vi "run.vi"(8 "error in (no error)":errorcluster, 11 "M1M3SAL in":refnum<class "M1M3SAL.lvclass">) -> (0 "error out":errorcluster, 3 "M1M3SAL out":refnum<class "M1M3SAL.lvclass">)   [LabVIEW 2016, in "M1M3SupportCommunicator.lvlib" / "M1M3SAL.lvclass"]
uses:
  M1M3SAL.lvclass
  M1M3SAL.lvclass/M1M3SAL.ctl
  UserEvents/UserEvents.lvclass/UserEvents.ctl
  DataTypes/Topics/EventSummaryState.ctl
  DataTypes/Topics/Parts/Timestamp.ctl
  DataTypes/Topics/Parts/SummaryStates.ctl
  DataTypes/Topics/Parts/CommandId.ctl
  DataTypes/Topics/CommandStart.ctl
  Commands/StartCommand/StartCommand.lvclass
  D:/Code/ts_M1M3Support/Commands/Command/Command.lvclass
  DataTypes/General/ProcessCommandEvent.ctl
  Commands/Command/Command.lvclass
  Commands/StartCommand/StartCommand.lvclass/StartCommand.ctl
  DataTypes/Topics/CommandEnable.ctl
  Commands/EnableCommand/EnableCommand.lvclass
  Commands/EnableCommand/EnableCommand.lvclass/EnableCommand.ctl
  DataTypes/Topics/CommandDisable.ctl
  Commands/DisableCommand/DisableCommand.lvclass
  Commands/DisableCommand/DisableCommand.lvclass/DisableCommand.ctl
  DataTypes/Topics/CommandStandby.ctl
  Commands/StandbyCommand/StandbyCommand.lvclass
  Commands/StandbyCommand/StandbyCommand.lvclass/StandbyCommand.ctl
  DataTypes/Topics/CommandExit.ctl
  Commands/ExitCommand/ExitCommand.lvclass
  Commands/ExitCommand/ExitCommand.lvclass/ExitCommand.ctl
  DataTypes/Topics/M1M3SupportTopics.lvlib
  DataTypes/General/M1M3SupportGeneral.lvlib
  UserEvents/UserEvents.lvclass
panel:
  out "Shutdown":bool
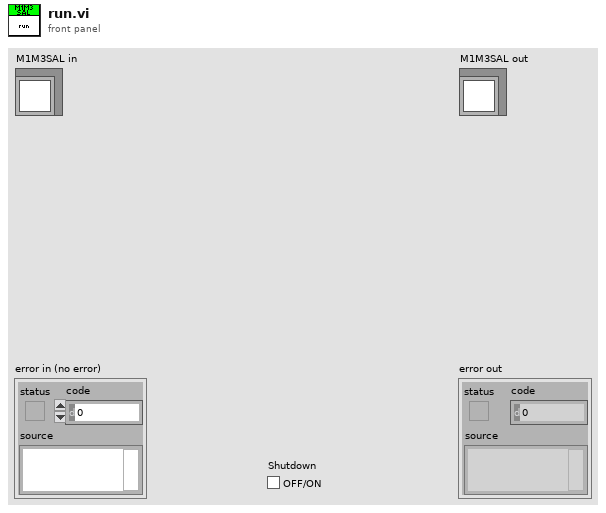
[diagram p1: front panel]
types:
  T1 = typedef "M1M3SupportTopics.lvlib/EventSummaryState.ctl" = cluster{"Timestamp":T2, "SummaryStates":T3}
  T2 = typedef "M1M3SupportTopics.lvlib/Timestamp.ctl" = dbl
  T3 = typedef "M1M3SupportTopics.lvlib/SummaryStates.ctl" = enum16{"OfflineState", "StandbyState", "DisabledState", "EnabledState", "FaultState"}
  T4 = typedef "M1M3SupportTopics.lvlib/CommandId.ctl" = i32
  T5 = typedef "M1M3SupportGeneral.lvlib/ProcessCommandEvent.ctl" = cluster{"Command":refnum<class "Command.lvclass">}
  T6 = typedef "M1M3SupportTopics.lvlib/CommandStart.ctl" = cluster{"CommandId":T4, "Start":bool, "SettingToApply":string}
  T7 = typedef "M1M3SupportTopics.lvlib/CommandEnable.ctl" = cluster{"CommandId":T4, "Enable":bool}
  T8 = typedef "M1M3SupportTopics.lvlib/CommandDisable.ctl" = cluster{"CommandId":T4, "Disable":bool}
  T9 = typedef "M1M3SupportTopics.lvlib/CommandStandby.ctl" = cluster{"CommandId":T4, "Standby":bool}
  T10 = typedef "M1M3SupportTopics.lvlib/CommandExit.ctl" = cluster{"CommandId":T4, "Exit":bool}
  T11 = typedef "M1M3SupportCommunicator.lvlib/Message.ctl" = cluster{"Header":T12, "Data":variant}
  T12 = typedef "M1M3SupportCommunicator.lvlib/MessageHeader.ctl" = cluster{"Type":T13, "Topic":T14, "Size":i32}
  T13 = typedef "M1M3SupportCommunicator.lvlib/MessageTypes.ctl" = enum8{"None", "PutSample", "GetNextSample", "LogEvent", "GetEvent", "IssueCommand", "CommandId", "WaitForCompletion", "AcceptCommand", "AckCommand"}
  T14 = typedef "M1M3SupportCommunicator.lvlib/MessageTopics.ctl" = enum8{"None", "ForceActuatorData", "MirrorForceData", "HardpointData", "AirData", "DynamicData", "FPGAData", "IMSData", "ForceActuatorStatus", "ElevationData", "HardpointStatus", "HardpointActuatorChase", "AirStatus", "ForceActuatorSafetyChecks", "ForceActuatorTest", "ActuatorBroadcastCounter", "StatusChecks", "CellChecks", "HardpointActuatorBreakaway", "RaiseMirrorComplete", "ILCCommunication", "ElevationAngleChecks", "DetailedState", "ServoLoops", "ForceActuatorInfo", "LowerMirrorComplete", "HardpointActuatorInfo", "SettingsApplied", "ErrorCode", "StartupChecks", "SummaryState", "SettingVersions", "ActuatorTestStatus", "AppliedSettingsMatchStart", "Enable", "EnterMaintenance", "Standby", "AbortLowerM1M3", "ApplyAberrationByForces", "ApplyAOSCorrectionByBendingModes", "ClearAOSCorrection", "Start", "RaiseM1M3", "TestForceActuator", "LowerM1M3", "ApplyAOSCorrectionByForces", "Disable", "ApplyAberationByBendingMode", "TestHardpoint", "ManipulateM1M3", "ClearAberration", "Exit", "TestAir", "AbortRaiseM1M3", "MoveHardpointActuators", "ExitMaintenance", "Shutdown"}
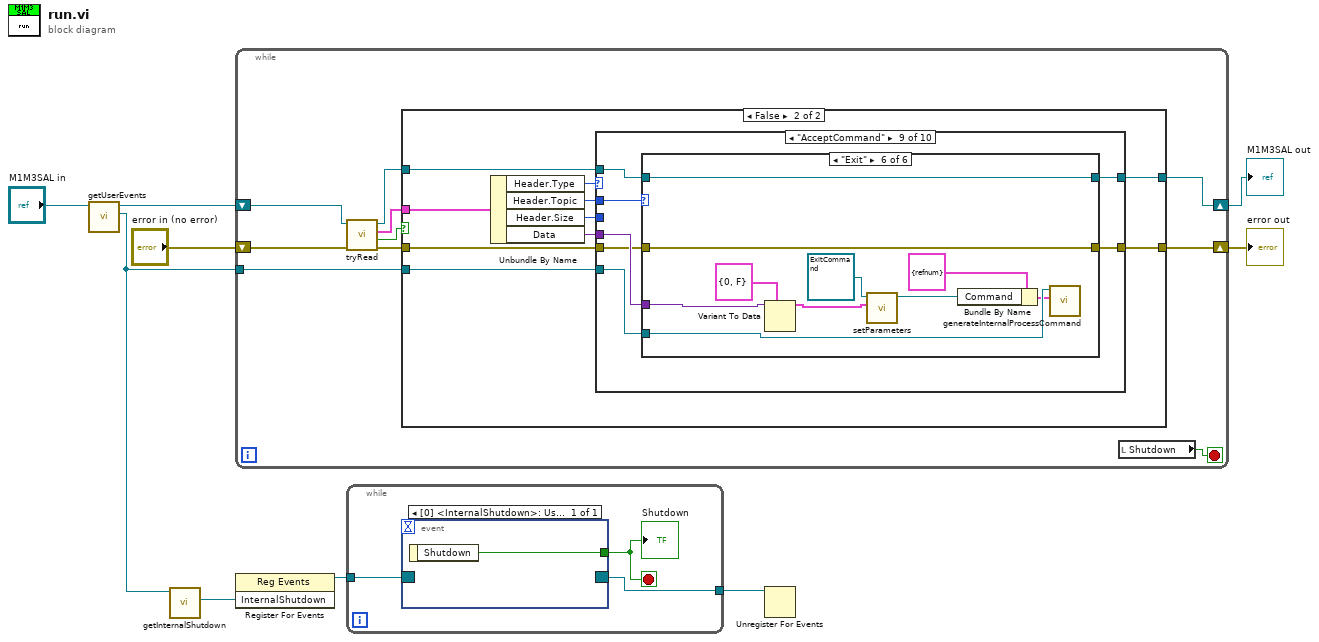
[diagram p0: block diagram]
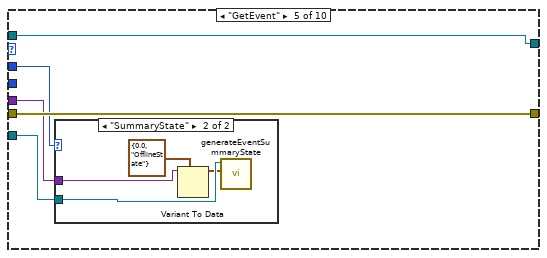
[diagram p7: hidden frame]
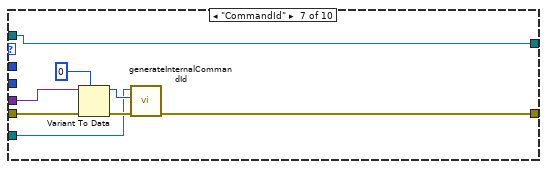
[diagram p10: hidden frame]
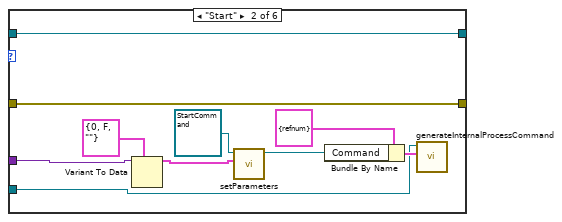
[diagram p13: hidden frame]
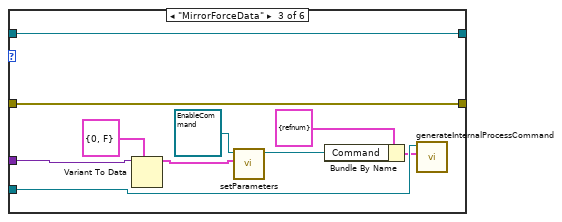
[diagram p14: hidden frame]
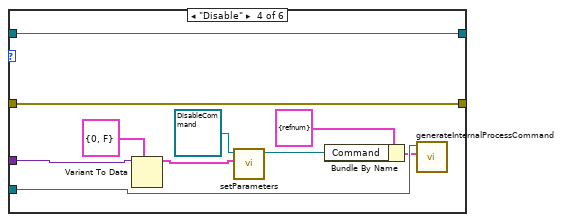
[diagram p15: hidden frame]
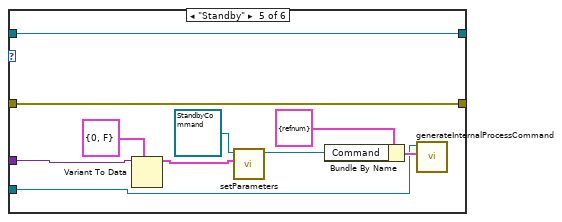
[diagram p16: hidden frame]
diagram:
  n1 = call "getUserEvents.vi"("M1M3SAL in"="M1M3SAL in") -> ("UserEvents"=w4:refnum<class "UserEvents.lvclass">, "M1M3SAL out"=w8:refnum<class "M1M3SAL.lvclass">)  [unwired: 9 in]
  n2 = call "getInternalShutdown.vi"("UserEvents in"=w4) -> ("InternalShutdown"=w3:refnum<user-event>)  [unwired: 9 in, 1 out]
  n3 = while {
    tunnel: w4 -> [w18]
    shift-right: [w15] -> w6
    shift-left: w8 -> [w17]
    shift-right: [w14] -> w5
    shift-left: "error in (no error)" -> [w13]
    stop <- w11 stop-if-true
    n4 = call "tryRead.vi"("error in (no error)"=w13, "M1M3SAL in"=w17) -> ("error out"=w12:errorcluster, "Timeout"=w10:bool, "Message"=w19:T11, "M1M3SAL out"=w16:refnum<class "M1M3SAL.lvclass">)  [unwired: 6 in]
    n5 = case shown="False" w10 {
      tunnel: w19 -> [_ w31]
      tunnel: w18 -> [_ w26]
      tunnel: w16 -> [w21 w25]
      tunnel: [w21 w24] -> w15
      tunnel: [w20 w23] -> w14
      tunnel: w12 -> [w20 w22]
      frame True {
      }
      frame False {
        n6 = Unbundle By Name(w31) -> ("Header.Type"=w30:T13, "Header.Topic"=w27:T14, "Header.Size"=w28:i32, "Data"=w29:variant)
        n7 = case shown="\"AcceptCommand\"" w30 {
          tunnel: w29 -> [_ _ _ _ w40 _ w57 _ w66 _]
          tunnel: w28 -> [_ _ _ _ _ _ _ _ _ _]
          tunnel: w27 -> [_ _ _ _ w41 _ _ _ w67 _]
          tunnel: w26 -> [_ _ _ _ w42 _ w51 _ w65 _]
          tunnel: w25 -> [w33 w35 w37 w39 w44 w50 w56 w60 w61 w121]
          tunnel: [w33 w35 w37 w39 w44 w50 w56 w60 w62 w121] -> w24
          tunnel: w22 -> [w32 w34 w36 w38 w43 w49 w55 w59 w64 w120]
          tunnel: [w32 w34 w36 w38 w43 w49 w52 w59 w63 w120] -> w23
          frame "None", Default {
          }
          frame "PutSample" {
          }
          frame "GetNextSample" {
          }
          frame "LogEvent" {
          }
          frame "GetEvent" {
            n8 = case shown="\"SummaryState\"" w41 {
              tunnel: w42 -> [_ w46]
              tunnel: w40 -> [_ w48]
              frame "None", Default {
              }
              frame "SummaryState" {
                n9 = Variant To Data(type=T1 {"Timestamp"=0.0, "SummaryStates"=enum."OfflineState"} ("EventSummaryState"), Variant=w48) -> (data=w45:T1)  [unwired: 1 in, 1 out]
                n10 = call "generateEventSummaryState.vi"("EventSummaryState"=w45, "UserEvents in"=w46) -> ()  [unwired: 8 in, 2 out]
              }
            }
          }
          frame "IssueCommand" {
          }
          frame "CommandId" {
            n11 = Variant To Data(error in=w55, type=T4 0 ("CommandId"), Variant=w57) -> (data=w54:T4, error out=w53:errorcluster)
            n12 = call "generateInternalCommandId.vi"("error in (no error)"=w53, "CommandId"=w54, "UserEvents in"=w51) -> ("error out"=w52:errorcluster)  [unwired: 7 in, 1 out]
          }
          frame "WaitForCompletion" {
          }
          frame "AcceptCommand" {
            n13 = case shown="\"Exit\"" w67 {
              tunnel: w66 -> [_ w79 w89 w99 w109 w119]
              tunnel: w65 -> [_ w70 w81 w91 w100 w111]
              tunnel: w64 -> [w69 w76 w86 w96 w106 w116]
              tunnel: [w69 w76 w86 w96 w106 w116] -> w63
              tunnel: [w68 w75 w85 w95 w105 w115] -> w62
              tunnel: w61 -> [w68 w75 w85 w95 w105 w115]
              frame "None", Default {
              }
              frame "Start" {
                n14 = Variant To Data(type=T6 {"CommandId"=0, "Start"=FALSE, "SettingToApply"=""} ("CommandStart"), Variant=w79) -> (data=w73:T6)  [unwired: 1 in, 1 out]
                n15 = call "setParameters.vi"("Parameters"=w73, "StartCommand in"=refnum<class "StartCommand.lvclass"> refnum ("StartCommand.lvclass")) -> ("StartCommand out"=w72:refnum<class "StartCommand.lvclass">)  [unwired: 9 in]
                n16 = Bundle By Name(cluster=T5 {"Command"=refnum} ("ProcessCommandEvent"), "Command"=w72) -> (w71:T5)
                n17 = call "generateInternalProcessCommand.vi"("ProcessCommandEvent"=w71, "UserEvents in"=w70) -> ()  [unwired: 8 in, 2 out]
              }
              frame "MirrorForceData" {
                n18 = Variant To Data(type=T7 {"CommandId"=0, "Enable"=FALSE} ("CommandEnable"), Variant=w89) -> (data=w83:T7)  [unwired: 1 in, 1 out]
                n19 = call "setParameters.vi"("Parameters"=w83, "EnableCommand in"=refnum<class "EnableCommand.lvclass"> refnum ("EnableCommand.lvclass")) -> ("EnableCommand out"=w82:refnum<class "EnableCommand.lvclass">)  [unwired: 9 in]
                n20 = Bundle By Name(cluster=T5 {"Command"=refnum} ("ProcessCommandEvent"), "Command"=w82) -> (w80:T5)
                n21 = call "generateInternalProcessCommand.vi"("ProcessCommandEvent"=w80, "UserEvents in"=w81) -> ()  [unwired: 8 in, 2 out]
              }
              frame "Disable" {
                n22 = Variant To Data(type=T8 {"CommandId"=0, "Disable"=FALSE} ("CommandDisable"), Variant=w99) -> (data=w93:T8)  [unwired: 1 in, 1 out]
                n23 = call "setParameters.vi"("Parameters"=w93, "DisableCommand in"=refnum<class "DisableCommand.lvclass"> refnum ("DisableCommand.lvclass")) -> ("DisableCommand out"=w92:refnum<class "DisableCommand.lvclass">)  [unwired: 9 in]
                n24 = Bundle By Name(cluster=T5 {"Command"=refnum} ("ProcessCommandEvent"), "Command"=w92) -> (w90:T5)
                n25 = call "generateInternalProcessCommand.vi"("ProcessCommandEvent"=w90, "UserEvents in"=w91) -> ()  [unwired: 8 in, 2 out]
              }
              frame "Standby" {
                n26 = Variant To Data(type=T9 {"CommandId"=0, "Standby"=FALSE} ("CommandStandby"), Variant=w109) -> (data=w103:T9)  [unwired: 1 in, 1 out]
                n27 = call "setParameters.vi"("Parameters"=w103, "StandbyCommand in"=refnum<class "StandbyCommand.lvclass"> refnum ("StandbyCommand.lvclass")) -> ("StandbyCommand out"=w102:refnum<class "StandbyCommand.lvclass">)  [unwired: 9 in]
                n28 = Bundle By Name(cluster=T5 {"Command"=refnum} ("ProcessCommandEvent"), "Command"=w102) -> (w101:T5)
                n29 = call "generateInternalProcessCommand.vi"("ProcessCommandEvent"=w101, "UserEvents in"=w100) -> ()  [unwired: 8 in, 2 out]
              }
              frame "Exit" {
                n30 = Variant To Data(type=T10 {"CommandId"=0, "Exit"=FALSE} ("CommandExit"), Variant=w119) -> (data=w113:T10)  [unwired: 1 in, 1 out]
                n31 = call "setParameters.vi"("Parameters"=w113, "ExitCommand in"=refnum<class "ExitCommand.lvclass"> refnum ("ExitCommand.lvclass")) -> ("ExitCommand out"=w112:refnum<class "ExitCommand.lvclass">)  [unwired: 9 in]
                n32 = Bundle By Name(cluster=T5 {"Command"=refnum} ("ProcessCommandEvent"), "Command"=w112) -> (w110:T5)
                n33 = call "generateInternalProcessCommand.vi"("ProcessCommandEvent"=w110, "UserEvents in"=w111) -> ()  [unwired: 8 in, 2 out]
              }
            }
          }
          frame "AckCommand" {
          }
        }
      }
    }
    n34 = local read "Shutdown"() -> (w11:bool)
  }
  "error out" <- w5
  "M1M3SAL out" <- w6
  n35 = register-events(w3) -> (reference out=w2:refnum<event-registration>)  [unwired: 2 in, 1 out]
  n36 = while {
    tunnel: w2 -> [w124]
    tunnel: [w122] -> w1
    stop <- w123 stop-if-true
    n37 = event shown="[0] <InternalShutdown>: User Event" {
      selector: w124 -> [_]
      dyn-events: [_] -> w122
      timeout: _ -> [_]
      tunnel: [w125] -> w123
      event User Event {
        n38 = event-data() -> ("Shutdown"=w125:bool)  [unwired: 1 in]
      }
    }
    "Shutdown" <- w123
  }
  n39 = Unregister For Events(event registration refnum=w1) -> ()  [unwired: 1 in, 1 out]
